vi "decodeMessage.vi"(8 "error in (no error)":errorcluster, 10 "MessageString":string, 11 "NetworkClient in":refnum<class "ImageStreamDecoder.lvclass">) -> (0 "error out":errorcluster, 2 "close":bool, 3 "NetworkClient out":refnum<class "ImageStreamDecoder.lvclass">)   [LabVIEW 2011, in "Hardware.lvlib" / "HWControllers.lvlib" / "ImageStreamDecoder.lvclass"]
uses:
  ImageStreamDecoder.lvclass
  <vilib>/xml/Load XML String.vi
  <vilib>/xml/Close Reference(Node).vi
  <vilib>/xml/NI_XML.lvlib
  Tools/Filing/FileSystem/FileSystem.lvclass
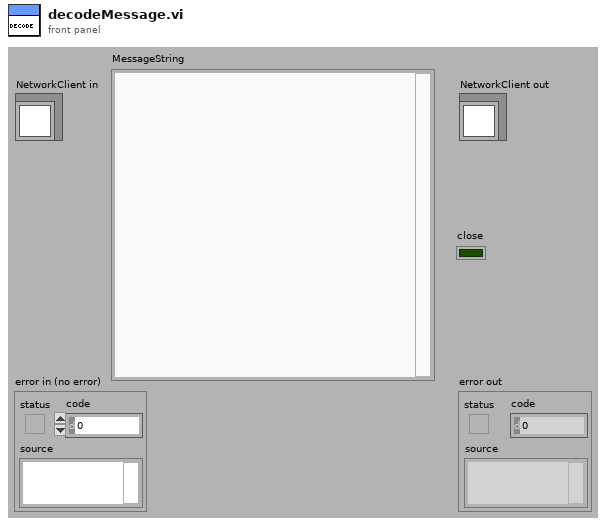
[diagram p1: front panel]
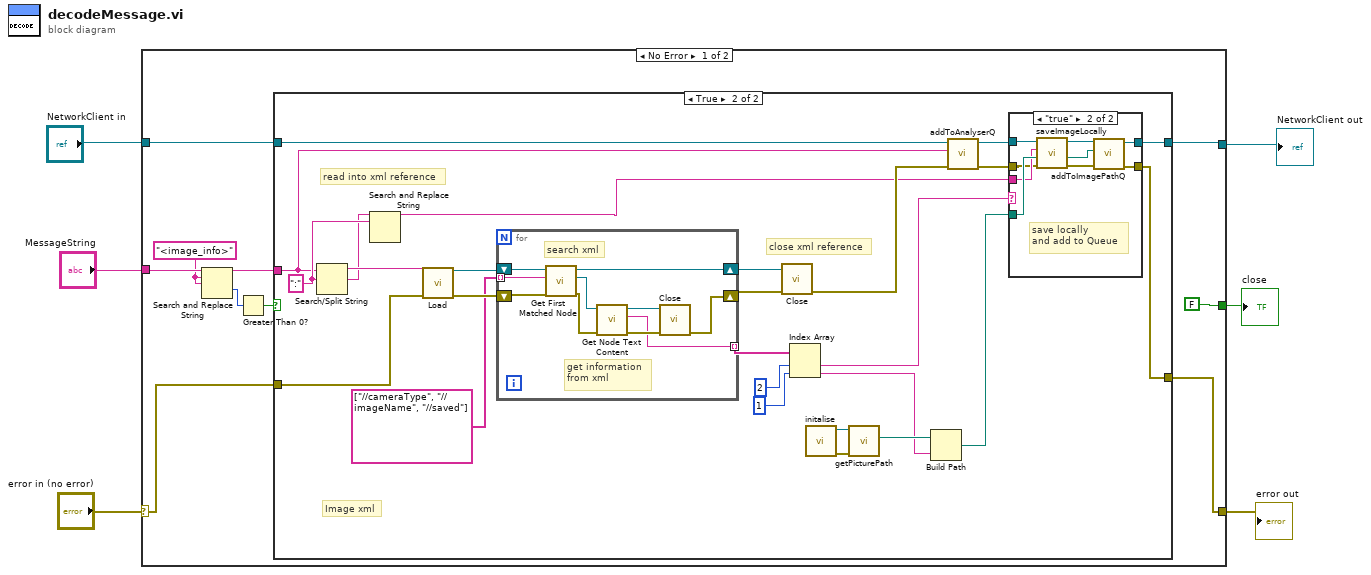
[diagram p0: block diagram]
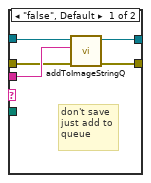
[diagram p3: hidden frame]
diagram:
  n1 = case shown="No Error" "error in (no error)" {
    selector: "error in (no error)" -> [w10 w69]
    tunnel: [w8 w70] -> w2
    tunnel: "NetworkClient in" -> [w9 w70]
    tunnel: [w7 w69] -> w5
    tunnel: "MessageString" -> [w15 _]
    tunnel: [FALSE _] -> w3
    frame No Error {
      w14 = "<image_info>"
      n2 = Search and Replace String(input string=w15, search string=w14, replace string=w14) -> (result string=w11:string, offset past replacement=w13:i32)  [unwired: 5 in, 2 out]
      n3 = Greater Than 0?(x=w13) -> (x > 0?=w12:bool)
      n4 = case shown="True" w12 {
        tunnel: w11 -> [_ w19]
        tunnel: w10 -> [w17 w44]
        tunnel: w9 -> [w18 w35]
        tunnel: [w18 w36] -> w8
        tunnel: [w17 w32] -> w7
        frame False {
          # "message not encoded properly"
        }
        frame True {
          w22 = ":"
          # "close xml reference"
          # "read into xml reference"
          # "Image xml"
          n5 = Search/Split String(string=w19, search string/char (-)=w22) -> (substring before match=w23:string, match + rest of string=w20:string)  [unwired: 1 in, 1 out]
          n6 = Search and Replace String(input string=w20, search string=w22) -> (result string=w21:string)  [unwired: 6 in, 3 out]
          n7 = call-poly <vilib>:"Load.vi"("XML string"=w23, "error in (no error)"=w44) -> ("DOM document out"=w43:refnum<k20>, "error out"=w42:errorcluster)  [unwired: 11 in, 1 out]
          n8 = for {
            tunnel: string[] ["//cameraType", "//imageName", "//saved"] -> [w66] mode=indexing
            shift-right: [w61] -> w40
            shift-left: w43 -> [w68]
            tunnel: [w60] -> w39 mode=indexing
            shift-right: [w59] -> w27
            shift-left: w42 -> [w67]
            # "search xml"
            # "get information\nfrom xml"
            n9 = call <vilib>:"Get First Matched Node.vi"("error in (no error)"=w67, "XPath expression"=w66, "node in"=w68) -> ("error out"=w65:errorcluster, "node result"=w64:refnum<k20>, "node out"=w61:refnum<k20>)  [unwired: 6 in]
            n10 = call <vilib>:"Get Node Text Content.vi"("error in (no error)"=w65, "node in"=w64) -> ("error out"=w63:errorcluster, "node text"=w60:string, "node out"=w62:refnum<k20>)  [unwired: 7 in]
            n11 = call-poly <vilib>:"Close.vi"("error in (no error)"=w63, "node"=w62) -> ("error out"=w59:errorcluster)  [unwired: 7 in]
          }
          n12 = call-poly <vilib>:"Close.vi"("error in (no error)"=w27, "node"=w40) -> ("error out"=w34:errorcluster)  [unwired: 7 in]
          n13 = Index Array(array=w39, index #1=2, index #2=1) -> (element #1=w31:string, element #2=w24:string)
          n14 = call "initalise.vi"() -> ("error out"=w28:errorcluster, "FileSystem out"=w29:refnum<class "FileSystem.lvclass">)  [unwired: 10 in]
          n15 = call "getPicturePath.vi"("error in (no error)"=w28, "FileSystem in"=w29) -> ("PicturePath"=w26:path)  [unwired: 7 in, 2 out]
          n16 = Build Path(base path=w26, name or relative path=w24) -> (appended path=w25:path)
          n17 = call "addToAnalyserQ.vi"("error in (no error)"=w34, "ImageString"=w19, "ImageStreamDecoder in"=w35) -> ("error out"=w33:errorcluster, "ImageStreamDecoder out"=w37:refnum<class "ImageStreamDecoder.lvclass">)  [unwired: 7 in]
          n18 = case shown="\"true\"" w31 {
            tunnel: w37 -> [w49 w56]
            tunnel: w21 -> [w47 w52]
            tunnel: [w48 w58] -> w36
            tunnel: w33 -> [w46 w51]
            tunnel: [w45 w57] -> w32
            tunnel: w25 -> [_ w53]
            frame "false", Default {
              # "don't save\njust add to\nqueue"
              n19 = call "addToImageStringQ.vi"("error in (no error)"=w46, "ImageString"=w47, "ImageStreamDecoder in"=w49) -> ("error out"=w45:errorcluster, "ImageStreamDecoder out"=w48:refnum<class "ImageStreamDecoder.lvclass">)  [unwired: 7 in]
            }
            frame "true" {
              # "save locally\nand add to Queue"
              n20 = call "saveImageLocally.vi"("error in (no error)"=w51, "Path"=w53, "ImageString"=w52, "ImageStreamDecoder in"=w56) -> ("error out"=w54:errorcluster, "Path out"=w50:path, "ImageStreamDecoder out"=w55:refnum<class "ImageStreamDecoder.lvclass">)  [unwired: 5 in]
              n21 = call "addToImagePathQ.vi"("error in (no error)"=w54, "ImagePath"=w50, "ImageStreamDecoder in"=w55) -> ("error out"=w57:errorcluster, "ImageStreamDecoder out"=w58:refnum<class "ImageStreamDecoder.lvclass">)  [unwired: 7 in]
            }
          }
        }
      }
    }
    frame Error {
    }
  }
  "error out" <- w5
  "close" <- w3
  "NetworkClient out" <- w2
